vi "And Operation (32).vi"(1 "X":bool[](array[boolean])=[FALSE, FALSE, FALSE, FALSE, FALSE, FALSE, FALSE, FALSE, FALSE, FALSE, FALSE, FALSE, FALSE, FALSE, FALSE, FALSE, FALSE, FALSE, FALSE, FALSE, FALSE, FALSE, FALSE, FALSE, FALSE, FALSE, FALSE, FALSE, FALSE, FALSE, FALSE, FALSE], 2 "Y":bool[](array[boolean])=[FALSE, FALSE, FALSE, FALSE, FALSE, FALSE, FALSE, FALSE, FALSE, FALSE, FALSE, FALSE, FALSE, FALSE, FALSE, FALSE, FALSE, FALSE, FALSE, FALSE, FALSE, FALSE, FALSE, FALSE, FALSE, FALSE, FALSE, FALSE, FALSE, FALSE, FALSE, FALSE]) -> (6 "X.and.Y?":bool[](array[boolean]))   [LabVIEW 2011]
doc: "This VI performs AND Operation on two 32 sized arrays"
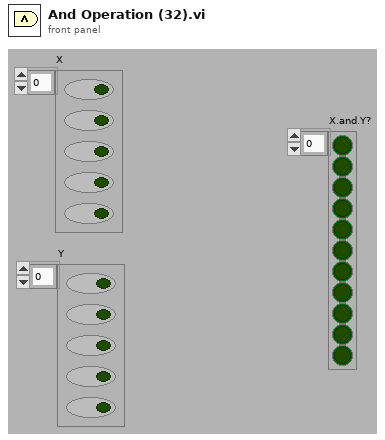
[diagram p1: front panel]
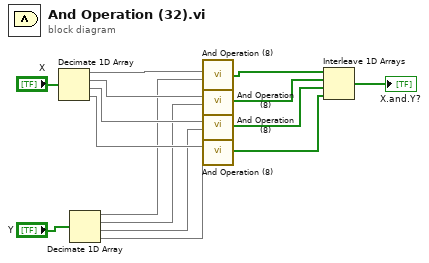
[diagram p0: block diagram]
diagram:
  n1 = Decimate 1D Array("X") -> (w14:bool[], w13:bool[], w12:bool[], w11:bool[])
  n2 = Decimate 1D Array("Y") -> (w9:bool[], w8:bool[], w7:bool[], w6:bool[])
  n3 = call <userlib>:"And Operation (8).vi"("Y"=w9, "X"=w14) -> ("X.and.Y?"=w5:bool[])  [unwired: 4 in]
  n4 = call <userlib>:"And Operation (8).vi"("Y"=w8, "X"=w13) -> ("X.and.Y?"=w4:bool[])  [unwired: 4 in]
  n5 = call <userlib>:"And Operation (8).vi"("Y"=w7, "X"=w12) -> ("X.and.Y?"=w3:bool[])  [unwired: 4 in]
  n6 = call <userlib>:"And Operation (8).vi"("Y"=w6, "X"=w11) -> ("X.and.Y?"=w2:bool[])  [unwired: 4 in]
  n7 = Interleave 1D Arrays(w5, w4, w3, w2) -> (→"X.and.Y?":bool[])
